vi "Reset Setpoints.vi"(8 "error in (no error)":errorcluster, 11 "Owlstone GEN-SYS in":refnum<class "Owlstone GEN-SYS.lvclass">) -> (0 "error out":errorcluster, 3 "Owlstone GEN-SYS out":refnum<class "Owlstone GEN-SYS.lvclass">)   [LabVIEW 2011, in "Owlstone GEN-SYS.lvclass"]
uses:
  Owlstone GEN-SYS.lvclass
  Owlstone GEN-SYS.lvclass/Owlstone GEN-SYS.ctl
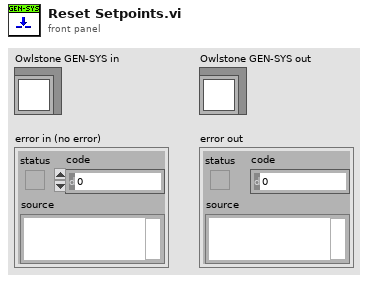
[diagram p1: front panel]
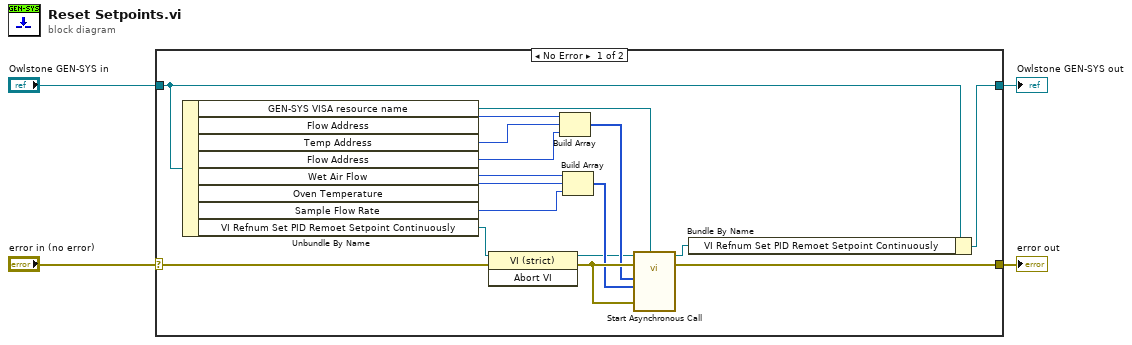
[diagram p0: block diagram]
diagram:
  n1 = case shown="No Error" "error in (no error)" {
    selector: "error in (no error)" -> [w6 w22]
    tunnel: [w21 w23] -> w4
    tunnel: [w20 w22] -> w3
    tunnel: "Owlstone GEN-SYS in" -> [w18 w23]
    frame No Error {
      n2 = Unbundle By Name(w18) -> ("GEN-SYS VISA resource name"=w8:refnum<visa-resource-name>, "Flow Address"=w9:u8, "Temp Address"=w10:u8, "Flow Address"=w11:u8, "Wet Air Flow"=w13:i32, "Oven Temperature"=w14:i32, "Sample Flow Rate"=w15:i32, "VI Refnum Set PID Remoet Setpoint Continuously"=w7:refnum<vi>)
      n3 = invoke class="VI (strict)" method="Abort VI"(reference=w7, error in=w6) -> (reference out=w5:refnum<vi>, error out=w17:errorcluster)  [unwired: 1 in, 1 out]
      n4 = Build Array(w9, w10, w11) -> (w12:u8[])
      n5 = Build Array(w13, w14, w15) -> (w16:i32[])
      n6 = call-by-ref "Start Asynchronous Call"(reference=w5, error in=w17, "VISA resource name"=w8, "error in"=w17, "Remote Setpoint"=w16, "Unit Addresses"=w12) -> (reference out=w19:refnum<vi>, error out=w20:errorcluster)  [unwired: 7 in, 1 out]
      n7 = Bundle By Name(cluster=w18, "VI Refnum Set PID Remoet Setpoint Continuously"=w19) -> (w21:refnum<class "Owlstone GEN-SYS.lvclass">)
    }
    frame Error {
    }
  }
  "Owlstone GEN-SYS out" <- w4
  "error out" <- w3
